vi "CheckName.vi"(8 "error in (no error)":errorcluster, 9 "FileName":string, 10 "ProjectName":string, 11 "SettingsFile in":refnum<class "SettingsFile.lvclass">) -> (0 "error out":errorcluster, 2 "Boolean":bool, 3 "SettingsFile out":refnum<class "SettingsFile.lvclass">)   [LabVIEW 2018, in "SettingsFile.lvclass"]
uses:
  SettingsFile.lvclass
  SettingsFile.lvclass/SettingsFile.ctl
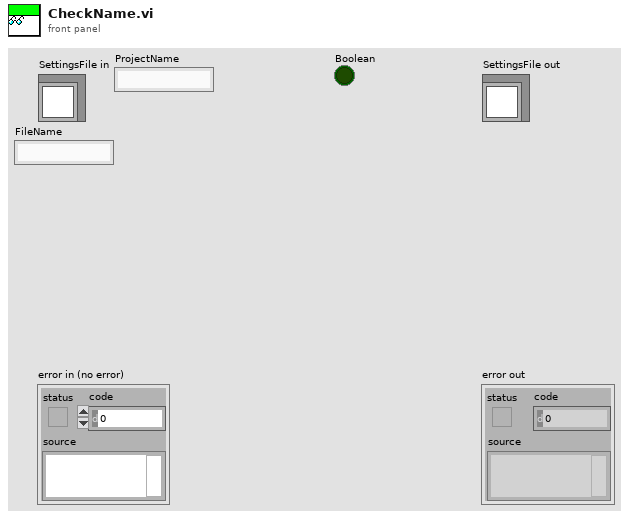
[diagram p1: front panel]
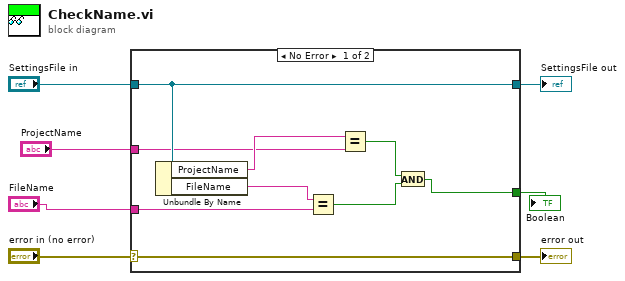
[diagram p0: block diagram]
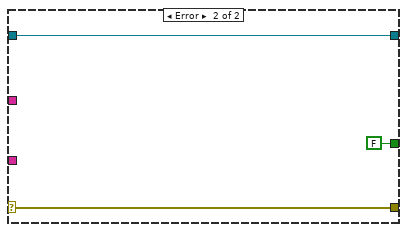
[diagram p2: hidden frame]
diagram:
  n1 = case shown="No Error" "error in (no error)" {
    selector: "error in (no error)" -> [w16 w18]
    tunnel: [w16 w18] -> w6
    tunnel: [w15 w19] -> w4
    tunnel: "SettingsFile in" -> [w15 w19]
    tunnel: "FileName" -> [w12 _]
    tunnel: "ProjectName" -> [w11 _]
    tunnel: [w8 FALSE] -> w1
    frame No Error {
      n2 = Unbundle By Name(w15) -> ("ProjectName"=w14:string, "FileName"=w13:string)
      n3 = Equal?(x=w13, y=w12) -> (x = y?=w9:bool)
      n4 = Equal?(x=w14, y=w11) -> (x = y?=w10:bool)
      n5 = And(x=w10, y=w9) -> (x .and. y?=w8:bool)
    }
    frame Error {
    }
  }
  "error out" <- w6
  "SettingsFile out" <- w4
  "Boolean" <- w1
